vi "PDC-4 Torque.vi"() -> ()   [LabVIEW 2021]
uses:
  Nanotec_PDC-4 Lib/typedef/prog_state.ctl
panel:
  out "sub state":string
  out "State":string
  out "Torque %":dbl
  out "Max Current\nmA":dbl format="%.2f"
  out "Current\nmA":dbl format="%.2f"
  in  "Max Torque\nNm":dbl
  in  "Write":T1={"Data (dec)"=0, FALSE, "Index"="``", "Sub-Index"="\u0000", "Data-Size (in Byte)"=1} {"Data-Size (in Byte)" min=1 max=4 step=1 format="%x"; "Data (dec)" step=1}
  out "Torque\nNm":dbl format="%.2f"
  out "Runtime Error":errorcluster
  in  "Stop":bool
  in  "error in":errorcluster
  in  "ComPort":refnum<visa-resource-name>="COM1"
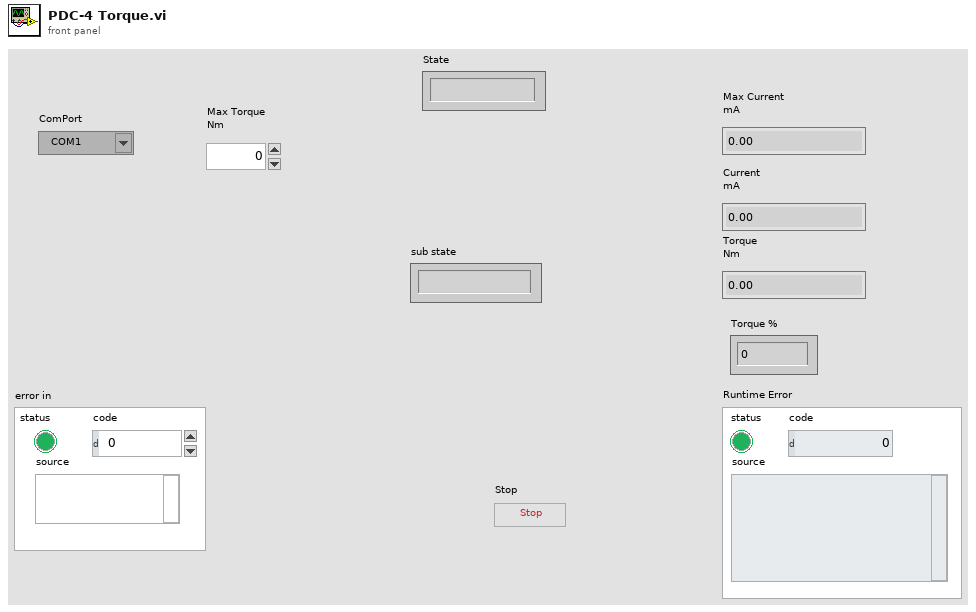
[diagram p1: front panel]
types:
  T1 = cluster{"Data (dec)":i32, bool, "Index":string, "Sub-Index":string, "Data-Size (in Byte)":u8}
  T2 = typedef "prog_state.ctl" = enum16{"init", "read", "write", "close", "error"}
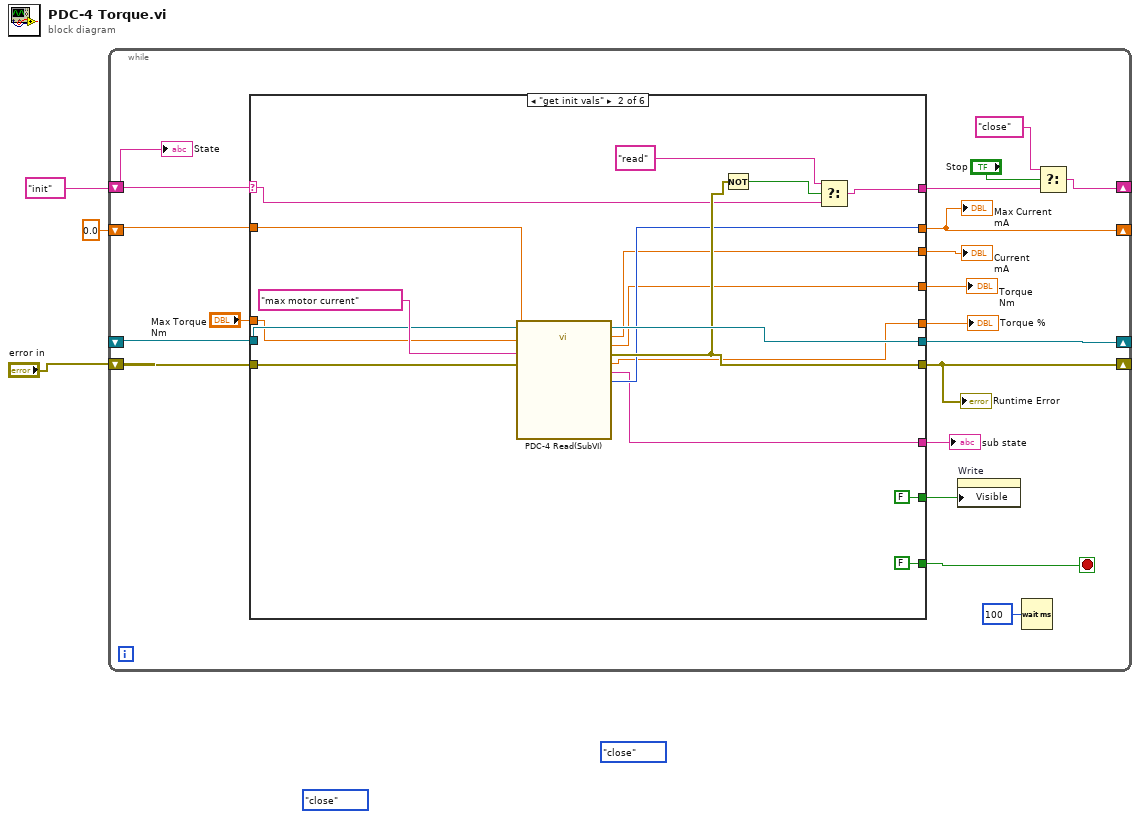
[diagram p0: block diagram]
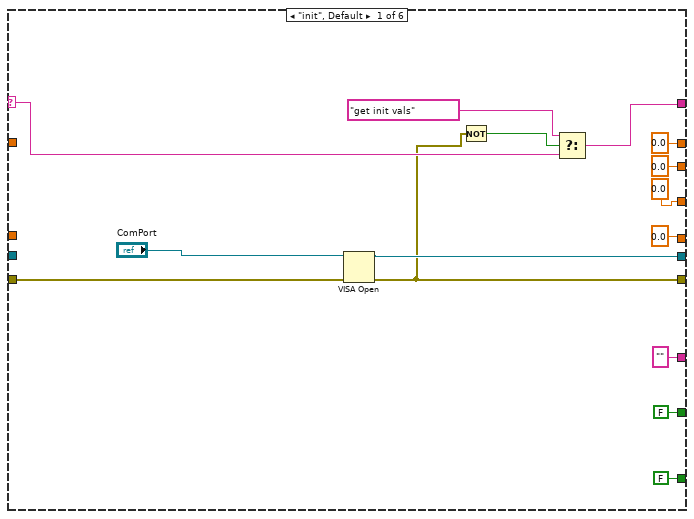
[diagram p2: hidden frame]
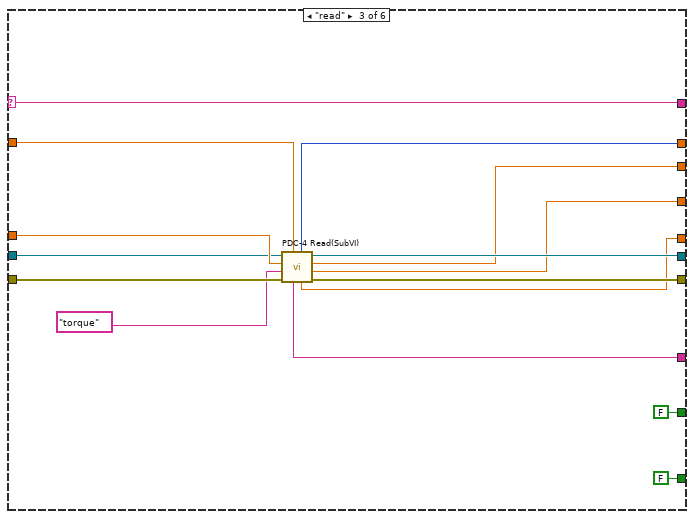
[diagram p3: hidden frame]
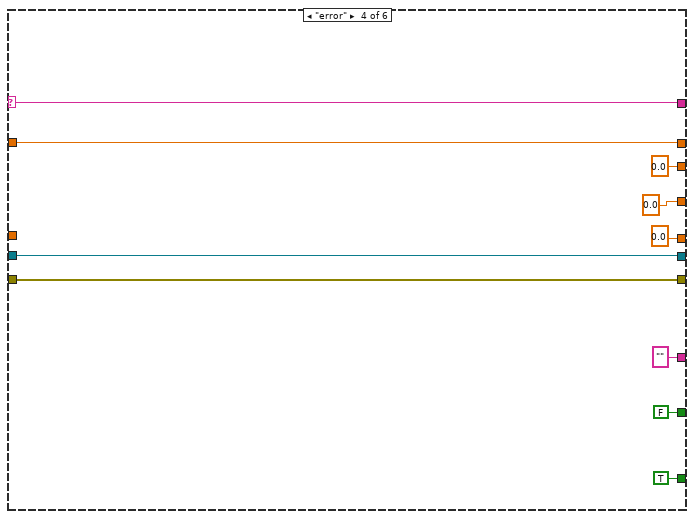
[diagram p4: hidden frame]
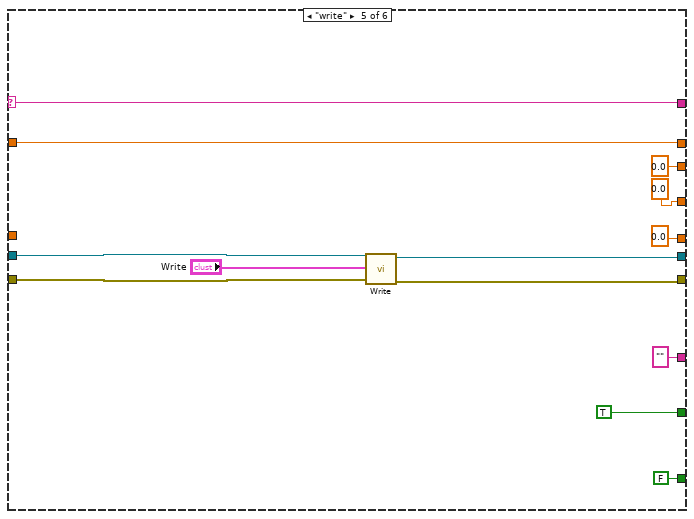
[diagram p5: hidden frame]
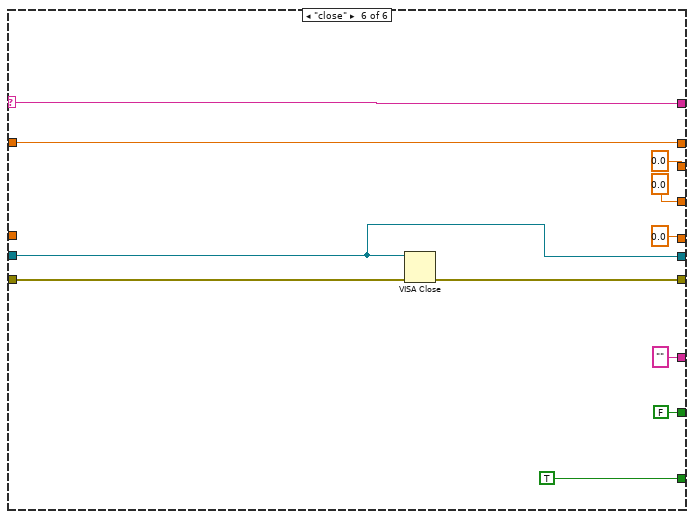
[diagram p6: hidden frame]
diagram:
  (unwired) prog_state."close" ("t")
  (unwired) prog_state."close" ("t")
  n1 = while {
    shift-right: [w19] -> _
    shift-left: "init" -> [w22]
    shift-right: [w17] -> _
    shift-left: _ -> [w9]
    shift-right: [w15] -> _
    shift-left: "error in" -> [w16]
    shift-right: [w13] -> _
    shift-left: 0.0 ("Motor Current mA") -> [w12]
    stop <- w18 stop-if-true
    n2 = case shown="\"get init vals\"" w22 {
      selector: w22 -> [w36 w46 w69 w80 w91 w103]
      tunnel: [w35 w45 w69 w80 w91 w103] -> w20
      tunnel: [FALSE FALSE FALSE TRUE FALSE TRUE] -> w18
      tunnel: [w34 w54 w64 w78 w86 w99] -> w17
      tunnel: [w26 w47 w63 w77 w85 w100] -> w15
      tunnel: w16 -> [w33 w53 w68 w77 w87 w101]
      tunnel: [FALSE ("Visible") FALSE ("Visible") FALSE ("Visible") FALSE ("Visible") TRUE ("Visible") FALSE ("Visible")] -> w14
      tunnel: [0.0 ("Motor Current mA") w42 w58 w79 w90 w97] -> w13
      tunnel: w12 -> [_ w52 w61 w79 w90 w97]
      tunnel: [0.0 ("Motor Current mA") w38 w62 0.0 ("Motor Current mA") 0.0 ("Motor Current mA") 0.0 ("Motor Current mA")] -> w11
      tunnel: "Max Torque\nNm" -> [_ w43 w66 _ _ _]
      tunnel: w9 -> [_ w44 w65 w78 w88 w99]
      tunnel: ["" ("state") w41 w59 "" ("state") "" ("state") "" ("state")] -> w6
      tunnel: [0.0 ("Torque %") w40 w56 0.0 ("Torque %") 0.0 ("Torque %") 0.0 ("Torque %")] -> w5
      tunnel: [0.0 ("Motor Torque Nm") w39 w57 0.0 ("Motor Torque Nm") 0.0 ("Motor Torque Nm") 0.0 ("Motor Torque Nm")] -> w4
      frame "init", Default {
        n3 = VISA Open(error in (no error)=w33, VISA resource name="ComPort") -> (VISA resource name=w34:refnum<visa-resource-name>, error out=w26:errorcluster)  [unwired: 3 in]
        n4 = Not(x=w26) -> (.not. x?=w27:bool)
        n5 = Select(t="get init vals", s=w27, f=w36) -> (s? t:f=w35:string)
      }
      frame "get init vals" {
        n6 = call "PDC-4 Read(SubVI).vi"("Max Current"=w52, "error in (no error)"=w53, "Data Req"="max motor current" ("String"), "Max Torque\nNm"=w43, "VISA Refnum in"=w44) -> ("error out"=w47:errorcluster, "Motor Torque Nm"=w39:dbl, "Motor Current mA"=w38:dbl, "VISA Refnum out"=w54:refnum<visa-resource-name>, "Torque %"=w40:dbl, "Max Motor Current mA"=w42:i32, "state"=w41:string)
        n7 = Not(x=w47) -> (.not. x?=w49:bool)
        n8 = Select(t="read", s=w49, f=w46) -> (s? t:f=w45:string)
      }
      frame "read" {
        n9 = call "PDC-4 Read(SubVI).vi"("Max Current"=w61, "error in (no error)"=w68, "Data Req"="torque" ("String"), "Max Torque\nNm"=w66, "VISA Refnum in"=w65) -> ("error out"=w63:errorcluster, "Motor Torque Nm"=w57:dbl, "Motor Current mA"=w62:dbl, "VISA Refnum out"=w64:refnum<visa-resource-name>, "Torque %"=w56:dbl, "Max Motor Current mA"=w58:i32, "state"=w59:string)
      }
      frame "error" {
      }
      frame "write" {
        n10 = call "Write.vi"("error in"=w87, "Write"="Write", "ComPort In"=w88) -> ("error out"=w85:errorcluster, "ComPort Out"=w86:refnum<visa-resource-name>)  [unwired: 7 in]
      }
      frame "close" {
        n11 = VISA Close(VISA resource name=w99, error in (no error)=w101) -> (error out=w100:errorcluster)
      }
    }
    "Runtime Error" <- w15
    "Torque\nNm" <- w4
    "Current\nmA" <- w11
    "Max Current\nmA" <- w13
    "Torque %" <- w5
    "sub state" <- w6
    n12 = property on="Write" class="Clust"("Visible"=w14) -> ()  [unwired: 2 in, 2 out]
    n13 = Wait (ms)(milliseconds to wait=u32 100) -> ()  [unwired: 1 out]
    n14 = Select(t="close", s="Stop", f=w20) -> (s? t:f=w19:string)
    "State" <- w22
  }
